vi "Check Digitizer Zeros.vi"(10 "# Consecutive Zeros Fault":i16=5000, 11 "DAQ Raw Data":T1=[0, 0, 0, 0, 0, 0, 0, 0, 0, 0, 0, 0, 0, 0, 0, 0, 0, 0, 0, 0, 0, 0, 0, 0, 0, 0, 0, 0, 0, 0, 0, 0, 0, 0, 0, 0, 0, 0]) -> (2 "DAQ Zero Fault":bool, 3 "DAQ Zero Fault Channel":bool[](array[boolean]))   [LabVIEW 2017]
doc: "Author: Scott Hannahs <sth@magnet.fsu.edu>\nCopyright 2018 Florida State University, All rights reserved."
uses:
  SCH Data Controls/SCH Raw Int Data.ctl
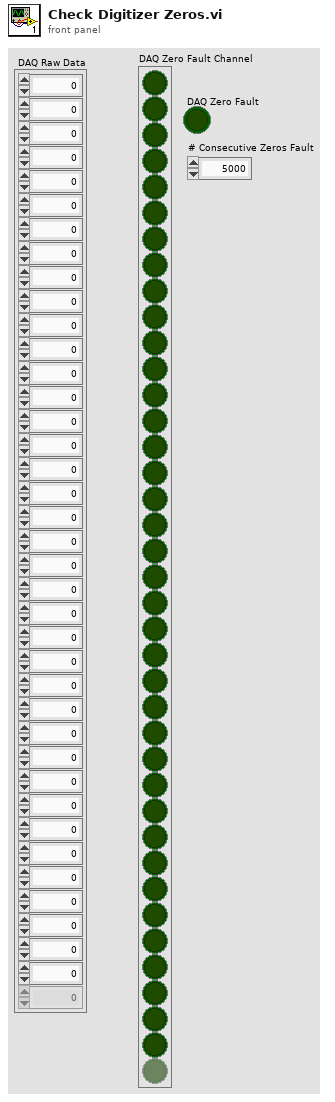
[diagram p1: front panel]
types:
  T1 = typedef "SCH Raw Int Data.ctl" = i16[]
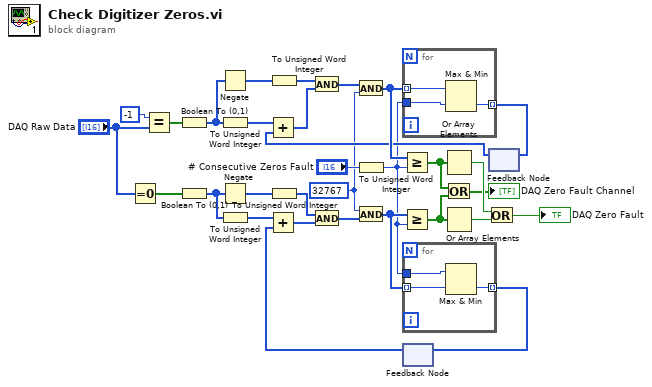
[diagram p0: block diagram]
diagram:
  w1 = u16 32767 ("# Consecutive Zeros Fault")
  n1 = Equal To 0?(x="DAQ Raw Data") -> (x = 0?=w31:bool[])
  n2 = Equal?(x=i16 -1, y="DAQ Raw Data") -> (x = y?=w12:bool[])
  n3 = Boolean To (0,1)(Boolean=w12) -> (0, 1=w18:i16[])
  n4 = Boolean To (0,1)(Boolean=w31) -> (0, 1=w25:i16[])
  n5 = Negate(x=w18) -> (-x=w14:i16[])
  n6 = To Unsigned Word Integer(number=w18) -> (unsigned 16bit integer=w17:u16[])
  n7 = Negate(x=w25) -> (-x=w29:i16[])
  n8 = To Unsigned Word Integer(number=w25) -> (unsigned 16bit integer=w26:u16[])
  n9 = To Unsigned Word Integer(number=w14) -> (unsigned 16bit integer=w19:u16[])
  n10 = To Unsigned Word Integer(number=w29) -> (unsigned 16bit integer=w24:u16[])
  n11 = To Unsigned Word Integer(number="# Consecutive Zeros Fault") -> (unsigned 16bit integer=w2:u16)
  n12 = feedback #1() -> (w30:u16[])  [unwired: 1 in]
  n13 = Add(x=w26, y=w30) -> (x+y=w28:u16[])
  n14 = And(x=w24, y=w28) -> (x .and. y?=w27:u16[])
  n15 = And(x=w1, y=w27) -> (x .and. y?=w22:u16[])
  n16 = Greater Or Equal?(x=w22, y=w2) -> (x >= y?=w4:bool[])
  n17 = for {
    tunnel: w22 -> [w32] mode=indexing
    tunnel: w2 -> [w33]
    tunnel: [w34] -> w23 mode=indexing
    n18 = Max & Min(x=w33, y=w32) -> (min(x,y)=w34:u16)  [unwired: 1 out]
  }
  n19 = feedback-in #1(w23) -> ()
  n20 = Or Array Elements(Boolean array=w4) -> (logical OR=w8:bool)
  n21 = feedback #2() -> (w13:u16[])  [unwired: 1 in]
  n22 = Add(x=w17, y=w13) -> (x+y=w15:u16[])
  n23 = And(x=w19, y=w15) -> (x .and. y?=w16:u16[])
  n24 = And(x=w16, y=w1) -> (x .and. y?=w21:u16[])
  n25 = Greater Or Equal?(x=w21, y=w2) -> (x >= y?=w5:bool[])
  n26 = for {
    tunnel: w21 -> [w35] mode=indexing
    tunnel: w2 -> [w36]
    tunnel: [w37] -> w20 mode=indexing
    n27 = Max & Min(x=w35, y=w36) -> (min(x,y)=w37:u16)  [unwired: 1 out]
  }
  n28 = Or Array Elements(Boolean array=w5) -> (logical OR=w7:bool)
  n29 = Or(x=w5, y=w4) -> (x .or. y?=→"DAQ Zero Fault Channel":bool[])
  n30 = Or(x=w7, y=w8) -> (x .or. y?=→"DAQ Zero Fault":bool)
  n31 = feedback-in #2(w20) -> ()
